vi "Tosca-Register TTL XControl Events.vi"(7 "Refs":refnum<vi>[](array[refnum]), 11 "error in (no error)":errorcluster) -> (8 "Event Registration Refnum":refnum<event-registration>, 10 "Events":T1[](array[typedef]), 15 "error out":errorcluster)   [LabVIEW 2015]
uses:
  TTLController XControl/Events.ctl
  TTLController XControl/Event Type.ctl
  TTLController XControl/Height Change.vi
  TTLController XControl/TTLController.xctl
panel:
  in  "temp":T2
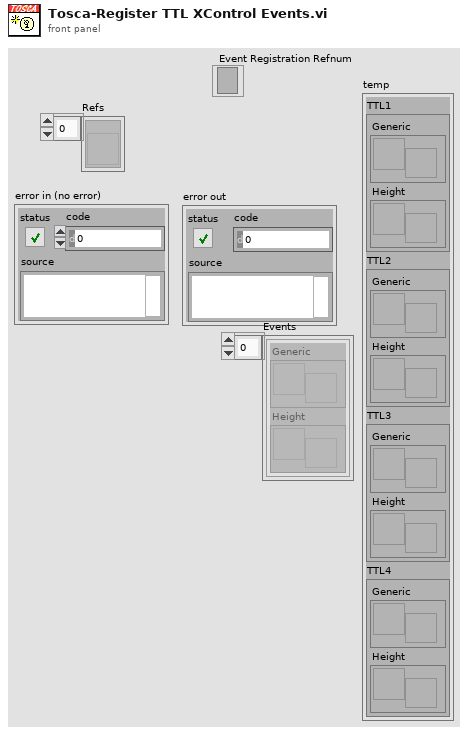
[diagram p1: front panel]
types:
  T1 = typedef "TTLController.xctl/Events.ctl" = cluster{"Generic":refnum<user-event>, "Height":refnum<user-event>}
  T2 = cluster{"TTL1":T1, "TTL2":T1, "TTL3":T1, "TTL4":T1}
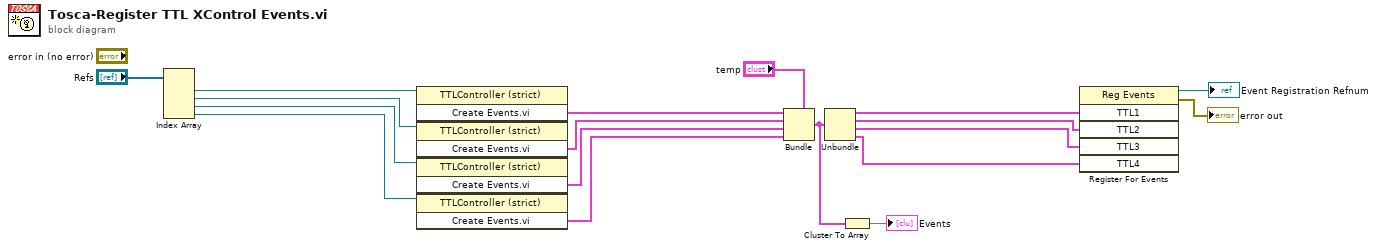
[diagram p0: block diagram]
diagram:
  n1 = Index Array(array="Refs") -> (element #1=w15:refnum<vi>, element #2=w12:refnum<vi>, element #3=w9:refnum<vi>, element #4=w6:refnum<vi>)  [unwired: 4 in]
  n2 = invoke class="TTLController (strict)" method="Create Events.vi"(reference=w15) -> ("Create Events.vi"=w14:T1)  [unwired: 2 in, 2 out]
  n3 = invoke class="TTLController (strict)" method="Create Events.vi"(reference=w12) -> ("Create Events.vi"=w11:T1)  [unwired: 2 in, 2 out]
  n4 = invoke class="TTLController (strict)" method="Create Events.vi"(reference=w9) -> ("Create Events.vi"=w8:T1)  [unwired: 2 in, 2 out]
  n5 = invoke class="TTLController (strict)" method="Create Events.vi"(reference=w6) -> ("Create Events.vi"=w5:T1)  [unwired: 2 in, 2 out]
  n6 = Bundle(cluster="temp", "TTL1"=w14, "TTL2"=w11, "TTL3"=w8, "TTL4"=w5) -> (w2:T2)
  n7 = Unbundle(w2) -> ("TTL1"=w13:T1, "TTL2"=w10:T1, "TTL3"=w7:T1, "TTL4"=w4:T1)
  n8 = Cluster To Array(cluster=w2) -> (array=→"Events":T1[])
  n9 = register-events(w13, w10, w7, w4) -> (reference out=→"Event Registration Refnum":refnum<event-registration>, error out=→"error out":errorcluster)  [unwired: 2 in]
